vi "Tacticbook_Init.vi"(0 "object in":refnum<class "Tacticbook.lvclass">, 5 "error in (no error)":errorcluster) -> (14 "object out":refnum<class "Tacticbook.lvclass">, 19 "error out":errorcluster)   [LabVIEW 2021, in "Tacticbook.lvclass"]
uses:
  Tacticbook.lvclass
  Tactic_class/Tactic.lvclass
  Tacticbook.lvclass/Tacticbook.ctl
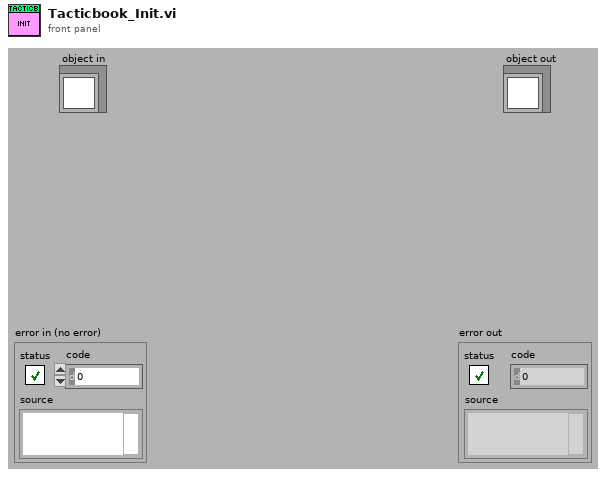
[diagram p1: front panel]
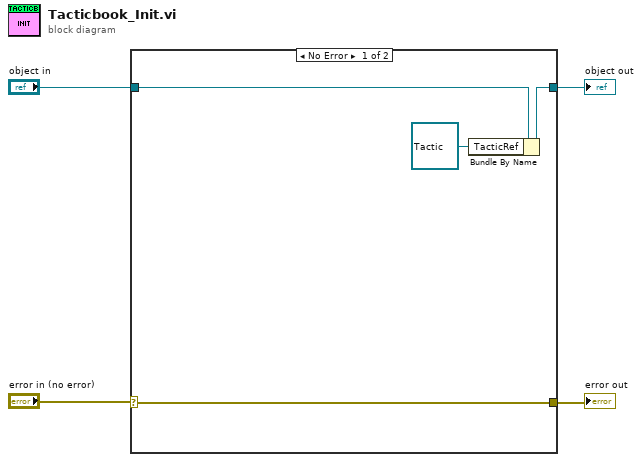
[diagram p0: block diagram]
diagram:
  n1 = case shown="No Error" "error in (no error)" {
    selector: "error in (no error)" -> [w6 w9]
    tunnel: "object in" -> [w8 w10]
    tunnel: [w7 w10] -> w3
    tunnel: [w6 w9] -> w1
    frame No Error {
      n2 = Bundle By Name(cluster=w8, "TacticRef"=refnum<class "Tactic.lvclass"> refnum) -> (w7:refnum<class "Tacticbook.lvclass">)
    }
    frame Error {
    }
  }
  "object out" <- w3
  "error out" <- w1
